vi "Read Config File Handle.vi"(11 "User Interface in":refnum<class "User Interface.lvclass">) -> (2 "Session Handle":T1, 3 "User Interface out":refnum<class "User Interface.lvclass">)   [LabVIEW 2016, in "_User Interface.lvlib" / "User Interface.lvclass"]
uses:
  User Interface.lvclass
  Configurations.lvclass
  Session Handle.ctl
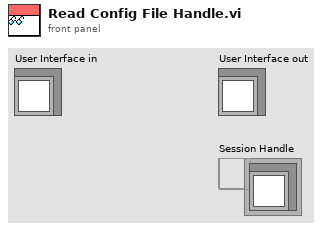
[diagram p1: front panel]
types:
  T1 = typedef "Configurations.lvlib/Configurations.lvclass/Session Handle.ctl" = refnum<data-value>
  T2 = typedef "_Configurations.lvlib/Configurations.lvclass/Session Handle.ctl" = refnum<data-value>
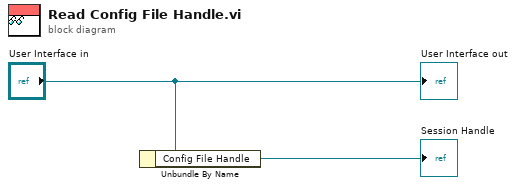
[diagram p0: block diagram]
diagram:
  n1 = Unbundle By Name("User Interface in") -> ("Config File Handle"=→"Session Handle":T2)
  "User Interface out" <- "User Interface in"
